vi "AnalogRead-8-9-10.vi"() -> (0 "Ch 10":dbl, 1 "Ch 9":dbl, 2 "Ch 8":dbl, 3 "N 10":u16, 4 "N 9":u32, 5 "N 8":u32)   [LabVIEW 2011]
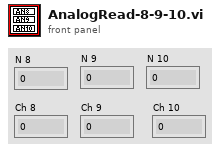
[diagram p1: front panel]
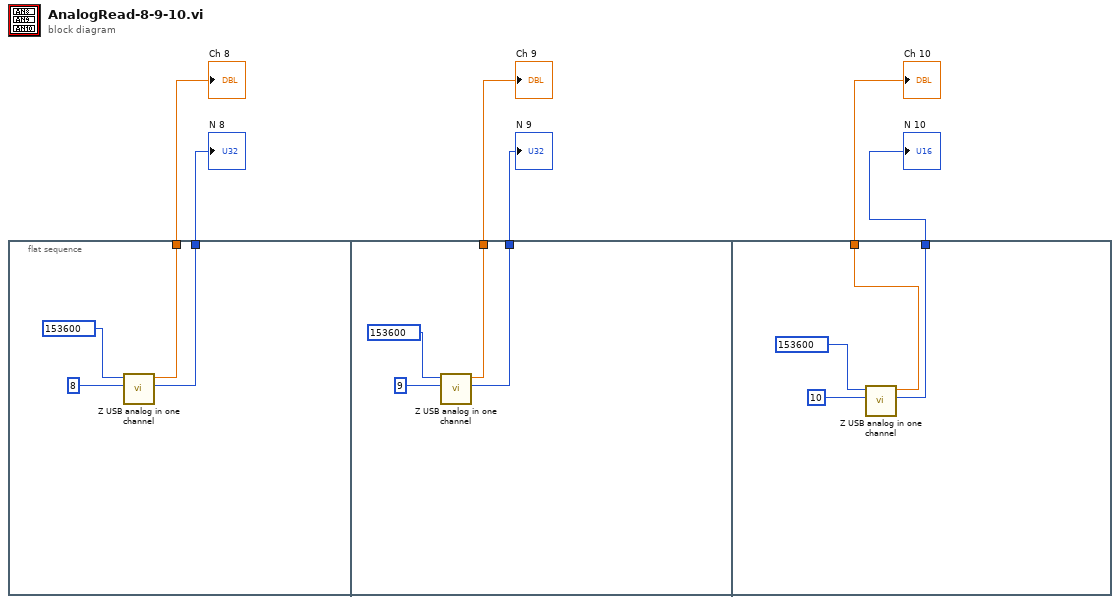
[diagram p0: block diagram]
diagram:
  n1 = flat-sequence {
    tunnel: [w10] -> w6
    tunnel: [w9] -> w3
    tunnel: [w14] -> w5
    tunnel: [w13] -> w2
    tunnel: [w18] -> w4
    tunnel: [w17] -> w1
    frame #0 {
      w8 = u32 153600 items=["9600"=9600, "19200"=19200, "38400"=38400, "76200"=76200, "153600"=153600, "307200"=307200, "614400"=614400, "1228800"=1228800] ("Baud Rate Asyn. Bit Bang")
      n2 = call "Z USB analog in one channel.vi"("Channel In"=u8 8, "Baud Rate Asyn. Bit Bang"=w8) -> ("N in"=w9:u32, "V in"=w10:dbl)  [unwired: 2 in, 2 out]
    }
    frame #1 {
      w12 = u32 153600 items=["9600"=9600, "19200"=19200, "38400"=38400, "76200"=76200, "153600"=153600, "307200"=307200, "614400"=614400, "1228800"=1228800] ("Baud Rate Asyn. Bit Bang")
      n3 = call "Z USB analog in one channel.vi"("Channel In"=u8 9, "Baud Rate Asyn. Bit Bang"=w12) -> ("N in"=w13:u32, "V in"=w14:dbl)  [unwired: 2 in, 2 out]
    }
    frame #2 {
      w16 = u32 153600 items=["9600"=9600, "19200"=19200, "38400"=38400, "76200"=76200, "153600"=153600, "307200"=307200, "614400"=614400, "1228800"=1228800] ("Baud Rate Asyn. Bit Bang")
      n4 = call "Z USB analog in one channel.vi"("Channel In"=u8 10, "Baud Rate Asyn. Bit Bang"=w16) -> ("N in"=w17:u32, "V in"=w18:dbl)  [unwired: 2 in, 2 out]
    }
  }
  "Ch 8" <- w6
  "Ch 9" <- w5
  "Ch 10" <- w4
  "N 8" <- w3
  "N 9" <- w2
  "N 10" <- w1
